vi "GUI.vi"() -> ()   [LabVIEW 2020]
uses:
  <vilib>/Instr/_visa.llb/VISA Configure Serial Port (Instr).vi
panel:
  out "Údaje z akcelerometra":cluster{dbl, dbl, i32}(graph)
  out "ODOSLANE HODNOTY":string
  in  "ODOSLAT \nHODNOTY":bool
  in  "Z [°]":dbl
  in  "X [°]":dbl
  in  "Y [°]":dbl
  out "Z [°]":i32
  out "Y [°]":i32
  out "X [°]":i32
  out "Údaje z enkóderov":cluster{dbl, dbl, i32}(graph)
  in  "stop":bool
  out "String":string
  out "error out 2":errorcluster
  out "error out":errorcluster
  # "NUMERICKÉ HODNOTY Z ENKÓDEROV"
  # "OVLÁDANIE"
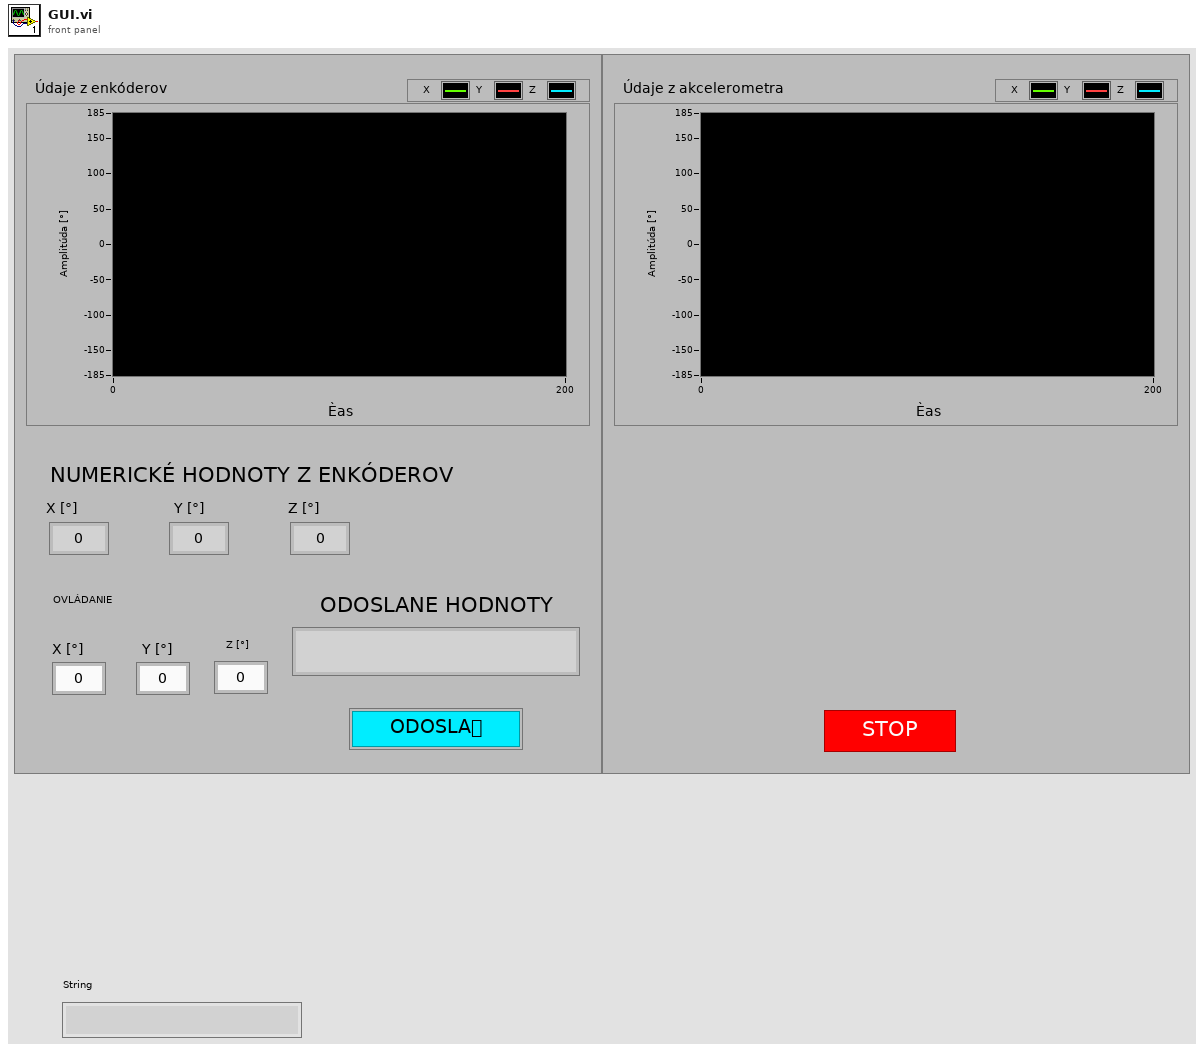
[diagram p1: front panel]
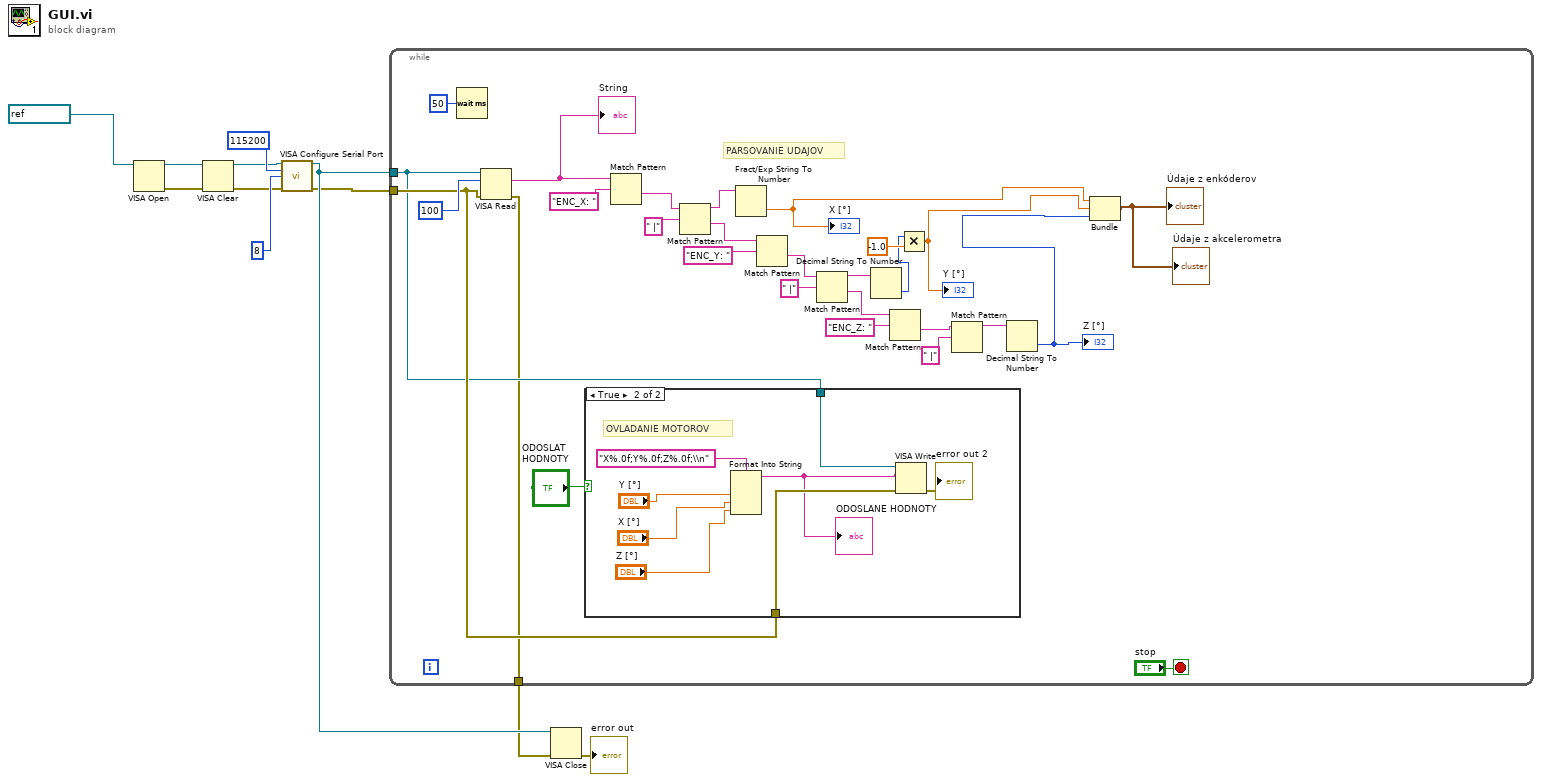
[diagram p0: block diagram]
diagram:
  n1 = VISA Open(VISA resource name=refnum<visa-resource-name> "COM7") -> (VISA resource name=w6:refnum<visa-resource-name>, error out=w4:errorcluster)  [unwired: 4 in]
  n2 = VISA Clear(VISA resource name=w6, error in (no error)=w4) -> (VISA resource name out=w5:refnum<visa-resource-name>, error out=w3:errorcluster)
  n3 = call-poly "VISA Configure Serial Port"("VISA resource name"=w5, "baud rate (9600)"=u32 115200, "data bits (8)"=u16 8, "error in (no error)"=w3) -> ("VISA resource name out"=w11:refnum<visa-resource-name>, "error out"=w10:errorcluster)  [unwired: 10 in]
  n4 = while {
    tunnel: w11 -> [w20]
    tunnel: w10 -> [w21]
    tunnel: [w19] -> w8
    stop <- "stop" stop-if-true
    # "PARSOVANIE UDAJOV"
    n5 = Wait (ms)(milliseconds to wait=u32 50) -> ()  [unwired: 1 out]
    n6 = VISA Read(VISA resource name=w20, byte count=u32 100, error in (no error)=w21) -> (read buffer=w37:string, error out=w19:errorcluster)  [unwired: 2 out]
    "String" <- w37
    n7 = case shown="True" "ODOSLAT \nHODNOTY" {
      tunnel: w20 -> [_ w43]
      tunnel: w21 -> [_ w42]
      frame False {
      }
      frame True {
        # "OVLADANIE MOTOROV"
        n8 = Format Into String(format string="X%.0f;Y%.0f;Z%.0f;\\n", "Y [°]", "X [°]", "Z [°]") -> (resulting string=w41:string)  [unwired: 2 in, 1 out]
        "ODOSLANE HODNOTY" <- w41
        n9 = VISA Write(VISA resource name=w43, write buffer=w41, error in (no error)=w42) -> (error out=→"error out 2":errorcluster)  [unwired: 2 out]
      }
    }
    n10 = Match Pattern(string=w37, regular expression="ENC_X: ") -> (after substring=w35:string)  [unwired: 1 in, 3 out]
    n11 = Match Pattern(string=w35, regular expression=" |") -> (before substring=w18:string, after substring=w25:string)  [unwired: 1 in, 2 out]
    n12 = Fract/Exp String To Number(string=w18) -> (number=w17:dbl)  [unwired: 3 in, 1 out]
    "X [°]" <- w17
    n13 = Match Pattern(string=w25, regular expression="ENC_Y: ") -> (after substring=w32:string)  [unwired: 1 in, 3 out]
    n14 = Match Pattern(string=w32, regular expression=" |") -> (before substring=w30:string, after substring=w24:string)  [unwired: 1 in, 2 out]
    n15 = Decimal String To Number(string=w30) -> (number=w12:i32)  [unwired: 2 in, 1 out]
    n16 = Match Pattern(string=w24, regular expression="ENC_Z: ") -> (after substring=w28:string)  [unwired: 1 in, 3 out]
    n17 = Multiply(x=w12, y=-1.0) -> (x*y=w13:dbl)
    "Y [°]" <- w13
    n18 = Match Pattern(string=w28, regular expression=" |") -> (before substring=w26:string)  [unwired: 1 in, 3 out]
    n19 = Decimal String To Number(string=w26) -> (number=w16:i32)  [unwired: 2 in, 1 out]
    "Z [°]" <- w16
    n20 = Bundle(w17, w13, w16) -> (→"Údaje z enkóderov" →"Údaje z akcelerometra":cluster{dbl, dbl, i32})  [unwired: 1 in]
  }
  n21 = VISA Close(VISA resource name=w11, error in (no error)=w8) -> (error out=→"error out":errorcluster)
